vi "Example Math 3.vi"() -> (3 "myvar":dbl caption="abs(x)")   [LabVIEW 2018]
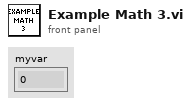
[diagram p1: front panel]
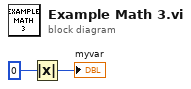
[diagram p0: block diagram]
diagram:
  n1 = Absolute Value(x=i16 0) -> (abs(x)=→"myvar":i16)
